vi "Coerce Input.vi"(0 "Max":dbl format="%.2f", 5 "Min":dbl format="%.2f", 9 "Input":dbl format="%.2f") -> (10 "Output":dbl format="%.2f")   [LabVIEW 2020]
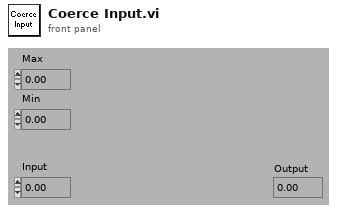
[diagram p1: front panel]
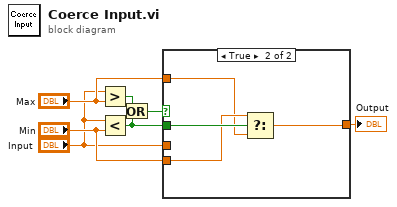
[diagram p0: block diagram]
diagram:
  n1 = Greater?(x="Input", y="Max") -> (0:w5:bool)
  n2 = Less?(x="Input", y="Min") -> (x < y?=w2:bool)
  n3 = Or(x=w5, y=w2) -> (x .or. y?=w4:bool)
  n4 = case shown="True" w4 {
    tunnel: "Input" -> [w8 _]
    tunnel: [w8 w9] -> w3
    tunnel: w2 -> [_ w12]
    tunnel: "Min" -> [_ w11]
    tunnel: "Max" -> [_ w10]
    frame False {
    }
    frame True {
      n5 = Select(t=w11, s=w12, f=w10) -> (s? t:f=w9:dbl)
    }
  }
  "Output" <- w3
